vi "String to Matrix (Norm).vi"(1 "Martix Dimension":i32, 2 "String":string) -> (0 "Output Matrix":T1)   [LabVIEW 2014]
uses:
  <vilib>/Analysis/Matrix/Datatypes/RealMatrix.ctl
  <vilib>/Analysis/Matrix/NI_Matrix.lvlib
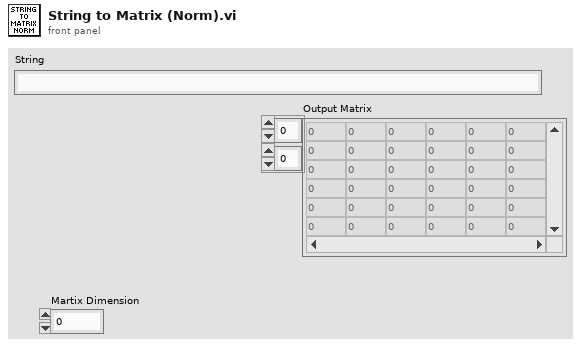
[diagram p1: front panel]
types:
  T1 = typedef "NI_Matrix.lvlib/RealMatrix.ctl" = dbl[][]
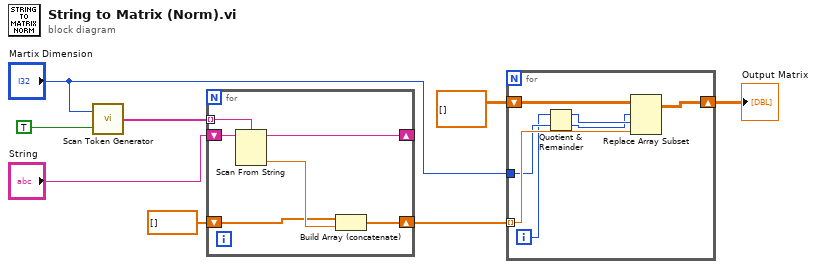
[diagram p0: block diagram]
diagram:
  n1 = call "Scan Token Generator.vi"("Matrix"=TRUE, "Martix Dimension"="Martix Dimension") -> ("Array"=w7:string[])
  n2 = for {
    tunnel: w7 -> [w12] mode=indexing
    shift-right: [w11] -> _
    shift-left: "String" -> [w14]
    shift-right: [w9] -> w6
    shift-left: dbl[] [] -> [w10]
    n3 = Scan From String(format string=w12, input string=w14) -> (remaining string=w11:string, output 1=w13:dbl)  [unwired: 3 in, 2 out]
    n4 = Build Array (concatenate)(w10, w13) -> (w9:dbl[])
  }
  n5 = for {
    tunnel: w6 -> [w21] mode=indexing
    tunnel: "Martix Dimension" -> [w20]
    shift-right: [w18] -> w2
    shift-left: T1 [] ("Empty Matrix") -> [w17]
    i -> [w19]
    n6 = Quotient & Remainder(x=w19, y=w20) -> (x-y*floor(x/y)=w16:i32, floor(x/y)=w15:i32)
    n7 = Replace Array Subset(array=w17, new element=w21, index (row)=w15, index (col)=w16) -> (w18:T1)
  }
  "Output Matrix" <- w2
